vi "Bundle Measurement Averages.vi"(0 "WT1800 Channel Group":i32, 1 "WT1800 Measurements":sgl[][](array[numeric]), 2 "DSA Measurements":sgl[][](array[numeric]), 5 "WT1800 Channels per Instrument":i32, 7 "Number of Functions":i32, 11 "Errors In":errorcluster[](array[cluster])) -> (4 "WT1800 Averages":T3 {"Vrms" format="%.3f"; "Irms" format="%.3f"; "Power" format="%.3f"; "Vpkpk" format="%.3f"; "Ipkpk" format="%.3f"}, 6 "DSA Averages":T1, 15 "Errors Out":errorcluster[](array[cluster]))   [LabVIEW 2021]
uses:
  Controls/WT1800 Measurements.ctl
  Controls/WT1800 Readings.ctl
  Controls/DSA Measurements.ctl
  Controls/DSA Readings.ctl
panel:
  in  "DSA Channels per Board":i32=2
  in  "DSA Channel Group":i32=1
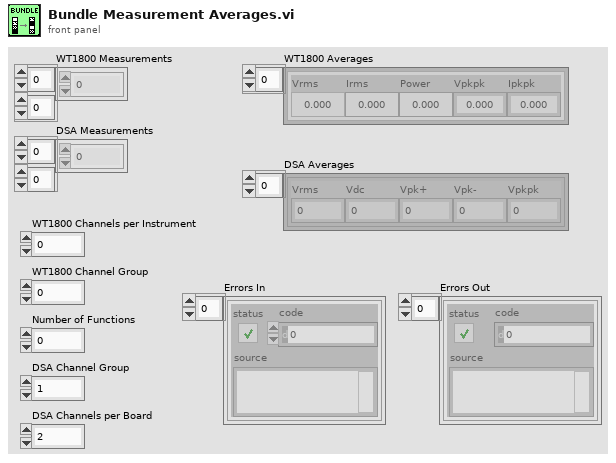
[diagram p1: front panel]
types:
  T1 = typedef "DSA Measurements.ctl" = T2[]
  T2 = typedef "DSA Readings.ctl" = cluster{"Vrms":sgl, "Vdc":sgl, "Vpk+":sgl, "Vpk-":sgl, "Vpkpk":sgl}
  T3 = typedef "WT1800 Measurements.ctl" = T4[]
  T4 = typedef "WT1800 Readings.ctl" = cluster{"Vrms":sgl, "Irms":sgl, "Power":sgl, "Vpkpk":sgl, "Ipkpk":sgl}
  T5 = cluster{"WT1800 Measurements[0]":sgl, "WT1800 Measurements[1]":sgl, "WT1800 Measurements[2]":sgl, "WT1800 Measurements[3]":sgl, "WT1800 Measurements[4]":sgl, "WT1800 Measurements[5]":sgl, "WT1800 Measurements[6]":sgl}
  T6 = cluster{"WT1800 Measurements[0]":sgl, "WT1800 Measurements[1]":sgl, "WT1800 Measurements[2]":sgl, "WT1800 Measurements[3]":sgl, "WT1800 Measurements[4]":sgl, "WT1800 Measurements[5]":sgl, "WT1800 Measurements[6]":sgl}[]
  T7 = cluster{"DSA Measurements[0]":sgl, "DSA Measurements[1]":sgl, "DSA Measurements[2]":sgl, "DSA Measurements[3]":sgl, "DSA Measurements[4]":sgl}
  T8 = cluster{"DSA Measurements[0]":sgl, "DSA Measurements[1]":sgl, "DSA Measurements[2]":sgl, "DSA Measurements[3]":sgl, "DSA Measurements[4]":sgl}[]
  T9 = cluster{sgl, sgl, "WT1800 Measurements[2]":sgl, sgl, sgl}
  T10 = cluster{sgl, "DSA Measurements[1]":sgl, "DSA Measurements[2]":sgl, "DSA Measurements[3]":sgl, "DSA Measurements[4]":sgl}
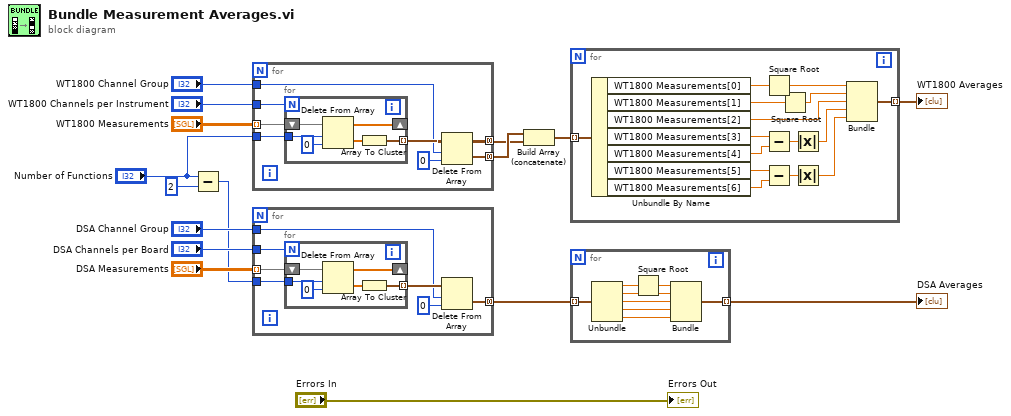
[diagram p0: block diagram]
diagram:
  n1 = Subtract(x="Number of Functions", y=2) -> (x-y=w8:i32)
  n2 = for {
    tunnel: [w24] -> w16 mode=concatenating
    tunnel: [w23] -> w15 mode=concatenating
    tunnel: "WT1800 Measurements" -> [w21] mode=indexing
    tunnel: "WT1800 Channel Group" -> [w20]
    tunnel: "Number of Functions" -> [w19]
    tunnel: "WT1800 Channels per Instrument" -> [w18]
    n3 = for {
      N: w18 -> [_]
      shift-right: [w29] -> _
      shift-left: w21 -> [w30]
      tunnel: w19 -> [w28]
      tunnel: [w27] -> w22 mode=indexing
      n4 = Delete From Array(array=w30, length=w28, index=0) -> (deleted portion=w26:sgl[], array with subset deleted=w29:sgl[])
      n5 = Array To Cluster(array=w26) -> (cluster=w27:T5)
    }
    n6 = Delete From Array(array=w22, length=w20, index=0) -> (deleted portion=w24:T6, array with subset deleted=w23:T6)
  }
  n7 = for {
    tunnel: [w37] -> w2 mode=concatenating
    tunnel: "DSA Measurements" -> [w35] mode=indexing
    tunnel: "DSA Channel Group" -> [w34]
    tunnel: w8 -> [w33]
    tunnel: "DSA Channels per Board" -> [w32]
    n8 = for {
      N: w32 -> [_]
      shift-right: [w42] -> _
      shift-left: w35 -> [w43]
      tunnel: w33 -> [w41]
      tunnel: [w40] -> w36 mode=indexing
      n9 = Delete From Array(array=w43, length=w41, index=0) -> (deleted portion=w39:sgl[], array with subset deleted=w42:sgl[])
      n10 = Array To Cluster(array=w39) -> (cluster=w40:T7)
    }
    n11 = Delete From Array(array=w36, length=w34, index=0) -> (deleted portion=w37:T8)  [unwired: 1 out]
  }
  n12 = Build Array (concatenate)(w16, w15) -> (w6:T6)
  n13 = for {
    tunnel: w6 -> [w58] mode=indexing
    tunnel: [w48] -> w4 mode=indexing
    n14 = Unbundle By Name(w58) -> ("WT1800 Measurements[0]"=w47:sgl, "WT1800 Measurements[1]"=w46:sgl, "WT1800 Measurements[2]"=w52:sgl, "WT1800 Measurements[3]"=w54:sgl, "WT1800 Measurements[4]"=w53:sgl, "WT1800 Measurements[5]"=w57:sgl, "WT1800 Measurements[6]"=w49:sgl)
    n15 = Square Root(x=w47) -> (sqrt(x)=w45:sgl)
    n16 = Subtract(x=w54, y=w53) -> (x-y=w55:sgl)
    n17 = Subtract(x=w57, y=w49) -> (x-y=w56:sgl)
    n18 = Square Root(x=w46) -> (sqrt(x)=w44:sgl)
    n19 = Absolute Value(x=w55) -> (abs(x)=w51:sgl)
    n20 = Absolute Value(x=w56) -> (abs(x)=w50:sgl)
    n21 = Bundle(w45, w44, "WT1800 Measurements[2]"=w52, w51, w50) -> (w48:T9)  [unwired: 1 in]
  }
  "WT1800 Averages" <- w4
  n22 = for {
    tunnel: w2 -> [w66] mode=indexing
    tunnel: [w64] -> w1 mode=indexing
    n23 = Unbundle(w66) -> ("DSA Measurements[0]"=w60:sgl, "DSA Measurements[1]"=w61:sgl, "DSA Measurements[2]"=w65:sgl, "DSA Measurements[3]"=w63:sgl, "DSA Measurements[4]"=w62:sgl)
    n24 = Square Root(x=w60) -> (sqrt(x)=w59:sgl)
    n25 = Bundle(w59, "DSA Measurements[1]"=w61, "DSA Measurements[2]"=w65, "DSA Measurements[3]"=w63, "DSA Measurements[4]"=w62) -> (w64:T10)  [unwired: 1 in]
  }
  "DSA Averages" <- w1
  "Errors Out" <- "Errors In"
